vi "Check Same Stream.vi"(8 "error in (no error)":errorcluster, 10 "Stream":refnum<class "Stream.lvclass">, 11 "Endpoint in":refnum<class "Endpoint.lvclass">) -> (0 "error out":errorcluster, 2 "Same?":bool, 3 "Endpoint out":refnum<class "Endpoint.lvclass">)   [LabVIEW 2020, in "Stream-Simple-Msg.lvlib" / "Endpoint.lvclass"]
uses:
  Endpoint.lvclass
  lv-stream/stream/Stream/Stream.lvclass
  Endpoint.lvclass/Endpoint.ctl
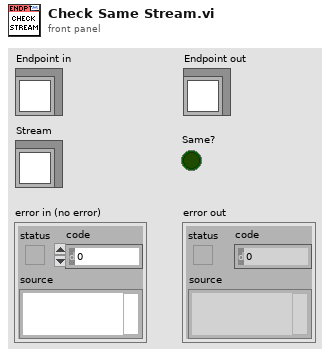
[diagram p1: front panel]
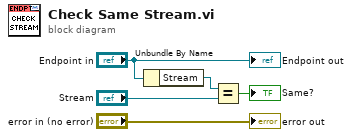
[diagram p0: block diagram]
diagram:
  n1 = Unbundle By Name("Endpoint in") -> ("Stream"=w2:refnum<class "Stream.lvclass">)
  n2 = Equal?(x=w2, y="Stream") -> (x = y?=→"Same?":bool)
  "error out" <- "error in (no error)"
  "Endpoint out" <- "Endpoint in"
